vi "InitializeDisplay.vi"(8 "error in (no error)":errorcluster, 11 "Display Queue in":refnum<queue>) -> (0 "error out":errorcluster, 3 "Display Queue out":refnum<queue>)   [LabVIEW 2017]
doc: "Enqueues the appropiate commands to the Display Queue for initializing the front panel of the ATM application."
uses:
  Downloads/ATM Simulator/Controls/DisplayControl.ctl
  controls/DisplayCommanda.ctl
  Downloads/ATM Simulator/Controls/EnableDisableCommand.ctl
  Downloads/ATM Simulator/Controls/UpdateMessageControl.ctl
  Downloads/ATM Simulator/Controls/UpdateMessageCommand.ctl
  Downloads/ATM Simulator/Controls/UpdateMenuCommand.ctl
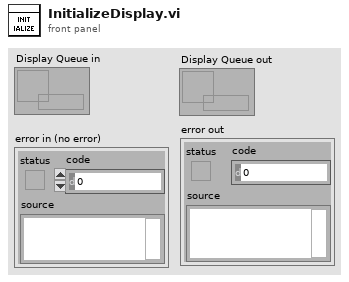
[diagram p1: front panel]
types:
  T1 = typedef "DisplayControl.ctl" = cluster{"Command":T2, "Data":variant}
  T2 = typedef "DisplayCommanda.ctl" = enum16{"Initialize", "Enable/Disable Controls", "FocusCursor", "UpdateMessage", "UpdateMenus", "FinishOperation", "Exit", "CleanUserInput"}
  T3 = typedef "UpdateMenuCommand.ctl" = enum16{"MainMenu", "NoMenu"}
  T4 = typedef "UpdateMessageControl.ctl" = cluster{"Command":T5, "Data":variant}
  T5 = typedef "UpdateMessageCommand.ctl" = enum16{"Welcome", "MainMenu", "AccountFailed", "SessionTerminate", "Deposit", "DepositComplete", "Withdrawal", "WithdrawalComplete", "WithdrawalFailed", "BalanceInquiry"}
  T6 = typedef "EnableDisableCommand.ctl" = enum16{"InitialSetup", "EnableUserInput", "DisableUserInput", "EnableMenus", "DisableMenus"}
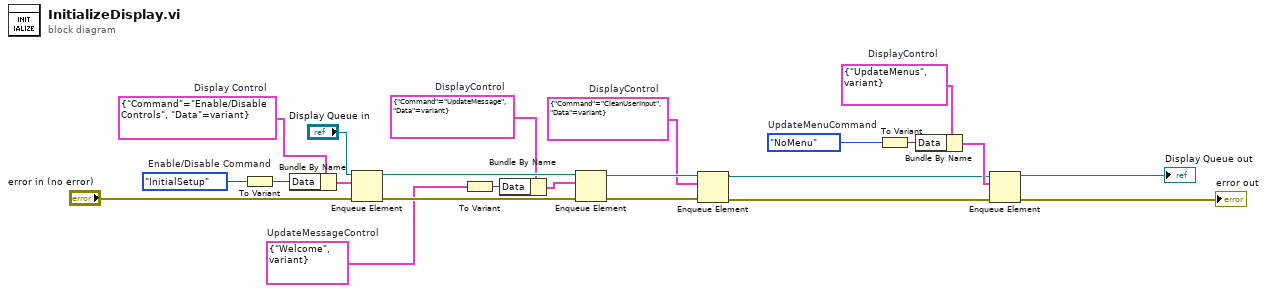
[diagram p0: block diagram]
diagram:
  w7 = T1 {"Command"=enum."UpdateMenus", "Data"=variant}  # DisplayControl
  w8 = UpdateMenuCommand."NoMenu"  # UpdateMenuCommand
  w9 = T1 {"Command"=enum."CleanUserInput", "Data"=variant}  # DisplayControl
  w12 = T4 {"Command"=enum."Welcome", "Data"=variant}  # UpdateMessageControl
  w13 = T1 {"Command"=enum."UpdateMessage", "Data"=variant}  # DisplayControl
  w22 = EnableDisableCommand."InitialSetup"  # Enable/Disable Command
  w20 = T1 {"Command"=enum."Enable/Disable Controls", "Data"=variant}  # Display Control
  n1 = To Variant(anything=w22) -> (Variant=w23:variant)
  n2 = Bundle By Name(cluster=w20, "Data"=w23) -> (w21:T1)
  n3 = Enqueue Element(queue="Display Queue in", element=w21, error in (no error)="error in (no error)") -> (queue out=w17:refnum<queue>, error out=w16:errorcluster)  [unwired: 1 in, 1 out]
  n4 = To Variant(anything=w12) -> (Variant=w15:variant)
  n5 = Bundle By Name(cluster=w13, "Data"=w15) -> (w14:T1)
  n6 = Enqueue Element(queue=w17, element=w14, error in (no error)=w16) -> (queue out=w10:refnum<queue>, error out=w11:errorcluster)  [unwired: 1 in, 1 out]
  n7 = Enqueue Element(queue=w10, element=w9, error in (no error)=w11) -> (queue out=w4:refnum<queue>, error out=w3:errorcluster)  [unwired: 1 in, 1 out]
  n8 = To Variant(anything=w8) -> (Variant=w5:variant)
  n9 = Bundle By Name(cluster=w7, "Data"=w5) -> (w6:T1)
  n10 = Enqueue Element(queue=w4, element=w6, error in (no error)=w3) -> (queue out=→"Display Queue out":refnum<queue>, error out=→"error out":errorcluster)  [unwired: 1 in, 1 out]
